vi "toNextYear.vi"(11 "Cron in":T1) -> (3 "Cron out":T1)   [LabVIEW 2013, in "openCron.lvlib" / "Cron.lvclass"]
uses:
  Cron.lvclass
  CronTime -- cluster.ctl
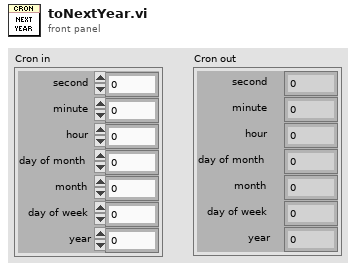
[diagram p1: front panel]
types:
  T1 = typedef "openCron.lvlib/Cron.lvclass/CronTime -- cluster.ctl" = cluster{"second":i32, "minute":i32, "hour":i32, "day of month":i32, "month":i32, "day of week":i32, "year":i32}
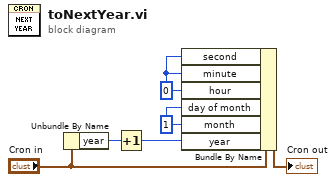
[diagram p0: block diagram]
diagram:
  w4 = 0 ("hour")
  w3 = 1 ("month")
  n1 = Unbundle By Name("Cron in") -> ("year"=w6:i32)
  n2 = Increment(x=w6) -> (x+1=w2:i32)
  n3 = Bundle By Name(cluster="Cron in", "second"=w4, "minute"=w4, "hour"=w4, "day of month"=w3, "month"=w3, "year"=w2) -> (→"Cron out":T1)
